vi "ExSimple.vi"() -> ()   [LabVIEW 2010]
panel:
  out "Intensity Graph":u16[][](graph)
  in  "Exposure":dbl=0.001 format="%.3f"
  in  "Close Compensation time ms 2":u32=8
  in  "Open Compensation time ms":u32=8
  in  "Temperature":dbl format="%.2f"
  out "error out":errorcluster
  in  "error in (no error)":errorcluster
  # "Note: for the Cascade and\nPhotonMax the open/close\n compensation should be 0"
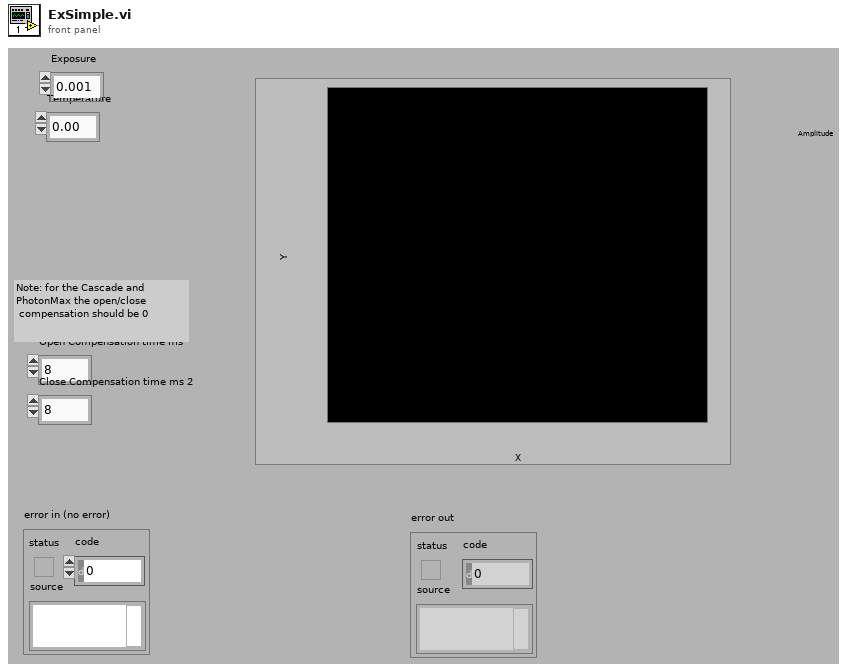
[diagram p1: front panel]
types:
  T1 = cluster{"Open Compensation time ms":u32, "Close Compensation time ms 2":u32}
  T2 = cluster{"Camera Handle":u32, "File Handle":u32, "Image Handle":u32}
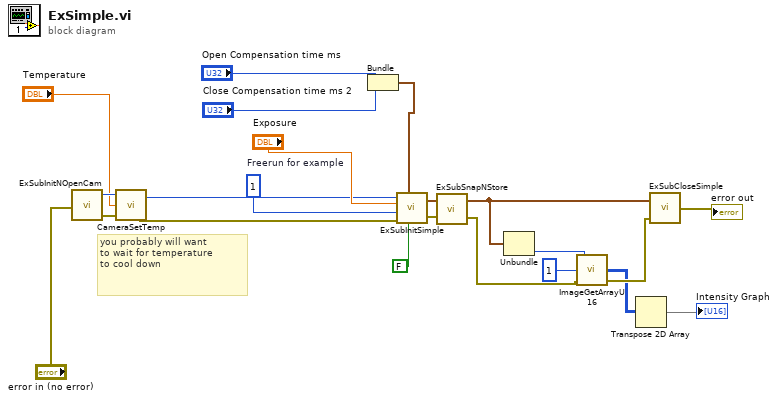
[diagram p0: block diagram]
diagram:
  w9 = 1  # Freerun for example
  # "you probably will want \nto wait for temperature \nto cool down"
  n1 = call "ExSubInitNOpenCam.vi"("error in (no error)"="error in (no error)") -> ("Camera Handle"=w20:u32, "error out"=w21:errorcluster)
  n2 = call <userlib>:"CameraSetTemp.vi"("error in (no error)"=w21, "Temperature"="Temperature", "Camera Handle"=w20) -> ("error out"=w15:errorcluster, "Camera Handle"=w8:u32)
  n3 = Bundle("Open Compensation time ms"="Open Compensation time ms", "Close Compensation time ms 2"="Close Compensation time ms 2") -> (w12:T1)  [unwired: 1 in]
  n4 = call "ExSubInitSimple.vi"("Intensifier"=FALSE, "Shutter Comp"=w12, "error in (no error)"=w15, "Triggering mode"=w9, "Exposure"="Exposure", "Camera Handle"=w8) -> ("error out"=w16:errorcluster, "Handles"=w17:cluster{"Camera":u32, "File":u32, "Image":u32})
  n5 = call "ExSubSnapNStore.vi"("error in (no error)"=w16, "Handle Cluster"=w17) -> ("error out"=w5:errorcluster, "Handle Cluster Out"=w7:T2)
  n6 = Unbundle(w7) -> ("Image Handle"=w6:u32)  [unwired: 2 out]
  n7 = call <userlib>:"ImageGetArrayU16.vi"("error in"=w5, "Z position"=1, "Image Handle"=w6) -> ("error out"=w4:errorcluster, "Array uint 16"=w2:u16[][])  [unwired: 1 out]
  n8 = Transpose 2D Array(2D array=w2) -> (transposed array=→"Intensity Graph":u16[][])
  n9 = call "ExSubCloseSimple.vi"("error in (no error)"=w4, "Handles In"=w7) -> ("error out"=→"error out":errorcluster)
